vi "Open Batch.vi"(6 "Batch Data 3":T2, 8 "error in (no error) 5":errorcluster, 9 "Primery key names":string[](array[string]), 10 "Primery key last values":string[](array[string]), 11 "Module Number  2":dbl=1.0) -> (0 "error out":errorcluster, 3 "Sucess ?":bool)   [LabVIEW 2015, in "Copy of Untitled Library 1.lvlib"]
uses:
  Copy of Untitled Library 1.lvlib
  Controls/Control 1.ctl
  Controls/Caller Queue Control .ctl
  Controls/Enum Constant.ctl
  <userlib>/origin_lib_main/db_interface/DB Operations Enum.ctl
  <userlib>/origin_lib_main/db_interface/DB Interface.lvlib
panel:
  in  "Cluster":T1
  in  "error in (no error) 6":errorcluster
  out "format string 2":string
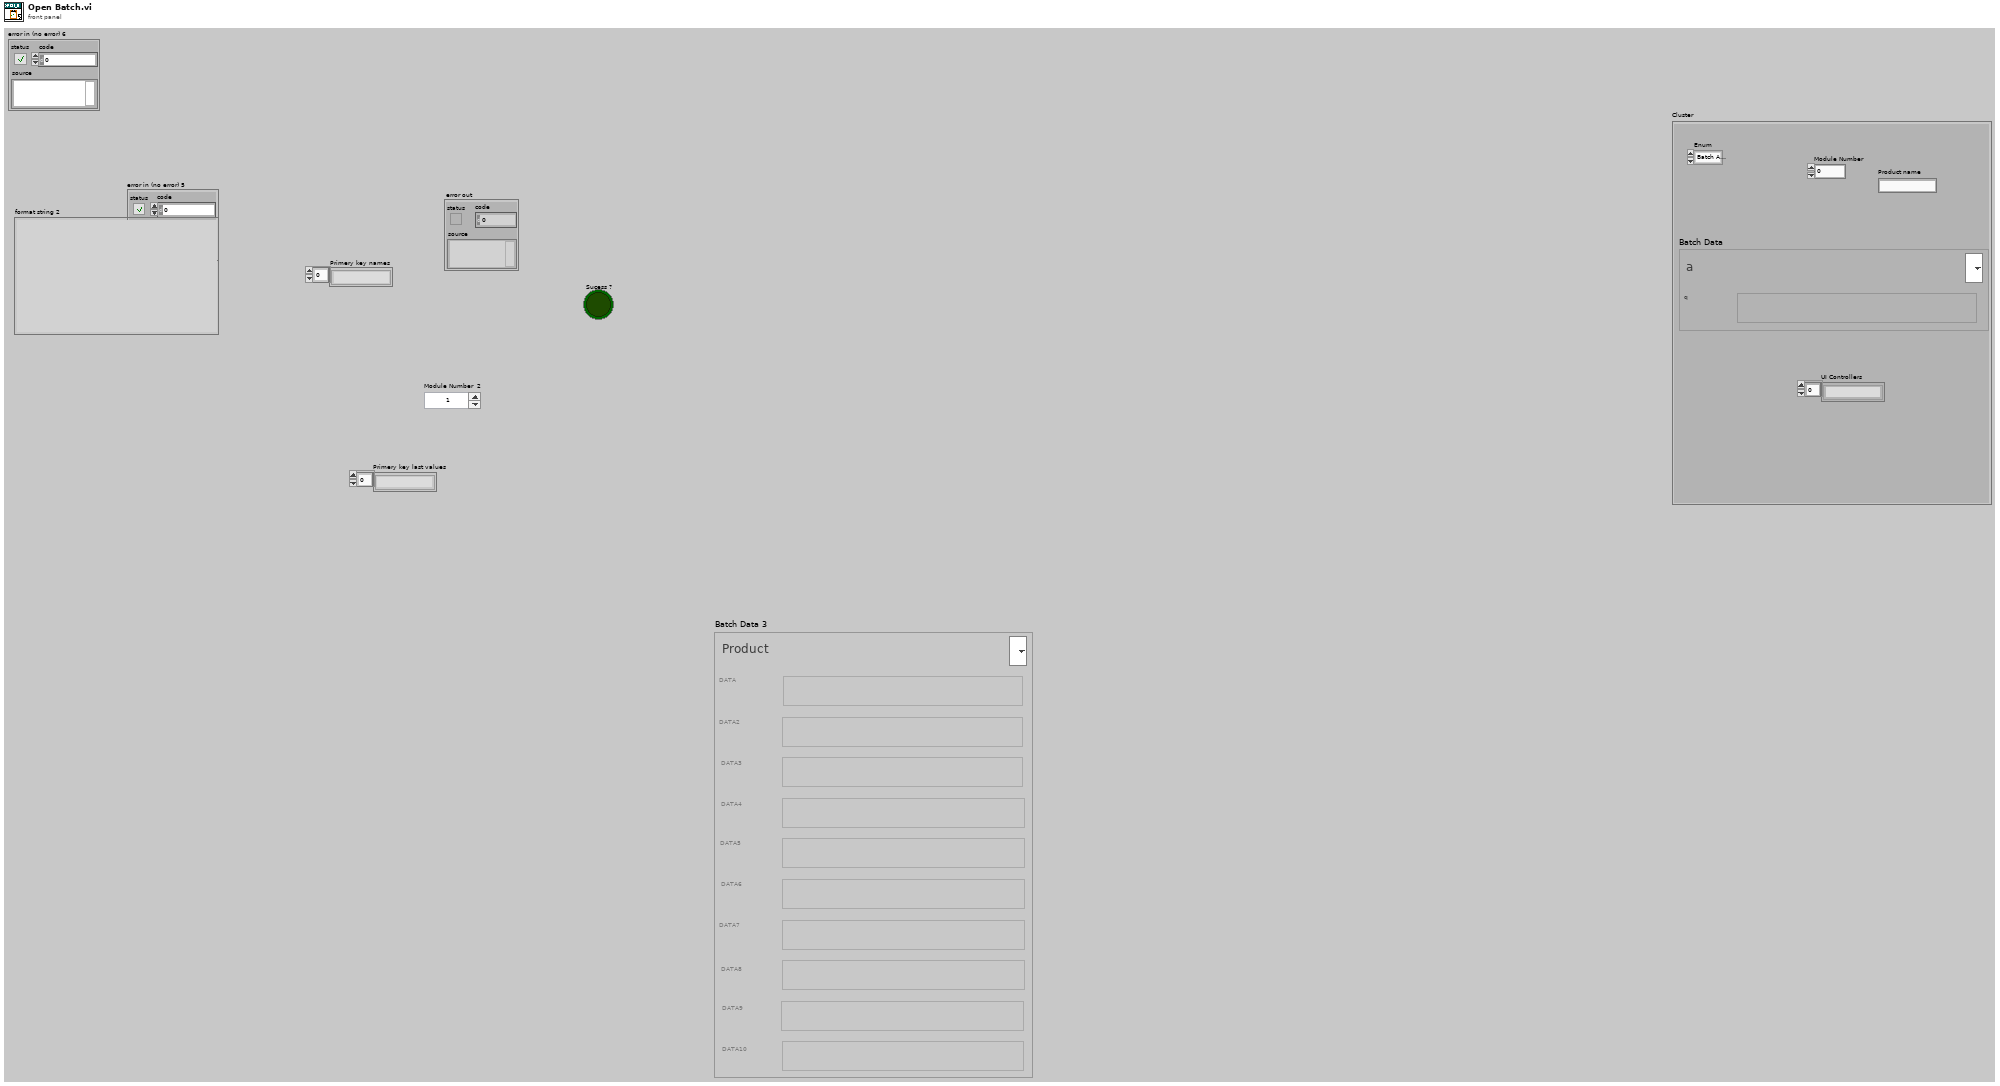
[diagram p1: front panel]
types:
  T1 = typedef "Caller Queue Control .ctl" = cluster{"Enum":enum16{"Batch Added", "Batch Deleted", "Batch Opened", "Batch Closed", "Batch Edited", "new Product Added", "Product deleted "}, "Batch Data 3":T2, "UI Controllers":string[], "Product name":string, "Module Number":dbl}
  T2 = typedef "Copy of Untitled Library 1.lvlib/Control 1.ctl" = cluster{"DATA":string, "DATA 2":string, "DATA 3":string, "DATA 4":string, "DATA 5":string, "DATA 6":string, "DATA 7":string, "DATA 8":string, "DATA 9":string, "DATA 10":string, "Product":string}
  T3 = typedef "DB Interface.lvlib/DB Operations Enum.ctl" = enum16{"Select", "Update", "Insert", "Delete", "Fetch SQL Query", "Execute SQL Query", "Drop Table", "List Tables"}
  T4 = typedef "Enum Constant.ctl" = enum16{"Init", "Read", "Write"}
  T5 = typedef "FGV Data.ctl" = T6[]
  T6 = typedef "FGV Cluster Data.ctl" = cluster{"Manual/Automatic":bool, "UI Controllers ":string[], "UI Primery Key ":dbl[], "Caller Queue & MSG":T7, "Module ID":dbl, "DB Reference In":T8, "Products Columns":string[], "Cluster":cluster{"Delete Product":enum8{"Enabled", "Disabled", "Disabled and Grayed Out"}, "Add Product ":enum8{"Enabled", "Disabled", "Disabled and Grayed Out"}, "EDIT BATCH":enum8{"Enabled", "Disabled", "Disabled and Grayed Out"}, "Open Batch ":enum8{"Enabled", "Disabled", "Disabled and Grayed Out"}, "Close Batch":enum8{"Enabled", "Disabled", "Disabled and Grayed Out"}, "Delete Batch":enum8{"Enabled", "Disabled", "Disabled and Grayed Out"}, "Add Batch ":enum8{"Enabled", "Disabled", "Disabled and Grayed Out"}}}
  T7 = typedef "Queue and Caller MSG.ctl" = cluster{"Caller Queue":refnum<queue>, "Caller MSG":string}
  T8 = typedef "NI_Database_API.lvlib/Conn ObjectReference.ctl" = refnum<k1>
  T9 = enum16{"Batch Added", "Batch Deleted", "Batch Opened", "Batch Closed", "Batch Edited", "new Product Added", "Product deleted "}
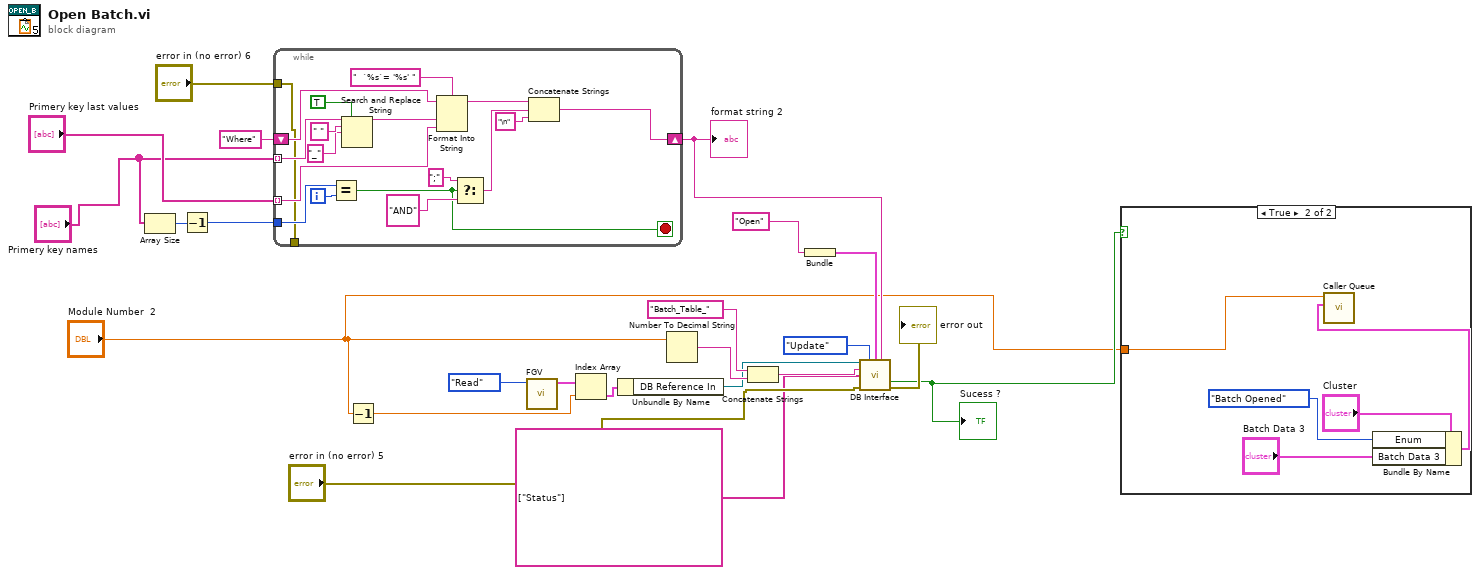
[diagram p0: block diagram]
diagram:
  n1 = Array Size(array="Primery key names") -> (size(s)=w8:i32)
  n2 = Decrement(x=w8) -> (x-1=w7:i32)
  n3 = while {
    shift-right: [w28] -> w3
    shift-left: "Where" ("format string") -> [w40]
    tunnel: w7 -> [w34]
    tunnel: "Primery key names" -> [w29] mode=indexing
    tunnel: "Primery key last values" -> [w26] mode=indexing
    tunnel: [w24] -> _
    tunnel: "error in (no error) 6" -> [w24]
    i -> [w35]
    stop <- w25 stop-if-true
    n4 = Equal?(x=w34, y=w35) -> (x = y?=w25:bool)
    n5 = Search and Replace String(replace all?=TRUE ("replace all? (F)"), input string=w29, search string=" ", replace string="_" ("replace string (\"\")")) -> (result string=w30:string)  [unwired: 4 in, 3 out]
    n6 = Format Into String(format string="  `%s`= '%s' ", initial string=w40, w30, w26) -> (resulting string=w39:string)  [unwired: 1 in, 1 out]
    n7 = Select(t=";", s=w25, f="AND") -> (s? t:f=w36:string)
    n8 = Concatenate Strings(w39, w36, "\n" ("string")) -> (w28:string)
  }
  "format string 2" <- w3
  n9 = Decrement(x="Module Number  2") -> (x-1=w16:dbl)
  n10 = call "FGV.vi"("Enum"=Enum_Constant."Read") -> ("Read Data"=w18:T5)  [unwired: 9 in, 1 out]
  n11 = Index Array(array=w18, index=w16) -> (element=w17:T6)
  n12 = Unbundle By Name(w17) -> ("DB Reference In"=w15:T8)
  n13 = Number To Decimal String(number="Module Number  2") -> (decimal integer string=w20:string)  [unwired: 1 in]
  n14 = Concatenate Strings("Batch_Table_" ("string"), w20) -> (w19:string)
  n15 = Bundle("condition"="Open") -> (w10:cluster{"condition":string})  [unwired: 1 in]
  n16 = call <userlib>:"DB Interface.vi"("DB Ref In"=w15, "Operation"=DB_Operations_Enum."Update", "data"=w10, "condition"=w3, "DB Table"=w19, "DB columns"=string[] ["Status"] ("element"), "error in (no error)"="error in (no error) 5") -> ("Sucess ?"=w2:bool, "error out"=→"error out":errorcluster)  [unwired: 5 in, 2 out]
  "Sucess ?" <- w2
  n17 = case shown="True" w2 {
    tunnel: "Module Number  2" -> [_ w44]
    frame False {
    }
    frame True {
      n18 = Bundle By Name(cluster="Cluster", "Enum"=T9."Batch Opened", "Batch Data 3"="Batch Data 3") -> (w42:T1)
      n19 = call "Caller Queue .vi"("Cluster"=w42, "Module Number  3"=w44) -> ()  [unwired: 9 in, 1 out]
    }
  }
